vi "Modify Pump Parameters.vi"(6 "timeout (1000 ms)":i32=1000, 7 "Query? (T)":bool=TRUE, 8 "error in (no error)":errorcluster, 10 "Parameters":T1={"Kc"=1.0, "Ti"=0.1, "Td"=0.0, "Min Speed"=0.0, "Max Speed"=100.0}, 11 "Pump in":refnum<class "Pump.lvclass">) -> (0 "error out":errorcluster, 2 "Parameters set":T1={"Kc"=1.0, "Ti"=0.1, "Td"=0.0, "Min Speed"=0.0, "Max Speed"=100.0}, 3 "Pump out":refnum<class "Pump.lvclass">, 4 "timed out?":bool)   [LabVIEW 2014, in "Pump.lvclass"]
doc: "For polynomial coefficients = [a, b, c]\nP(x) = a + b*(x^1) + c*(x^2)"
uses:
  Pump.lvclass
  Parameters - cluster.ctl
  Parameters Payload -- cluster.ctl
  Pump.lvclass/Pump.ctl
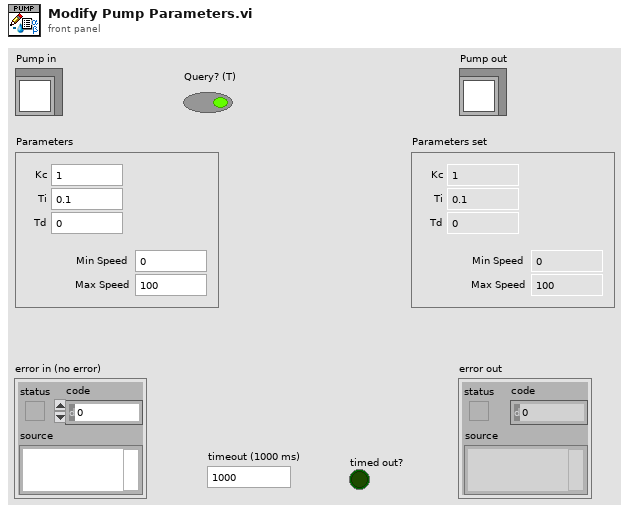
[diagram p1: front panel]
types:
  T1 = typedef "Pump.lvclass/Parameters - cluster.ctl" = cluster{"Kc":dbl, "Ti":dbl, "Td":dbl, "Min Speed":dbl, "Max Speed":dbl}
  T2 = typedef "Pump.lvclass/Parameters Payload -- cluster.ctl" = cluster{"Parameters":T1, "notifier":refnum<notifier>, "Query (T)":bool}
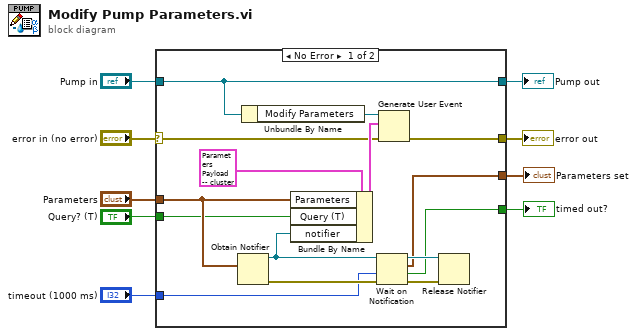
[diagram p0: block diagram]
diagram:
  n1 = case shown="No Error" "error in (no error)" {
    selector: "error in (no error)" -> [w16 w26]
    tunnel: [w15 w26] -> w8
    tunnel: [w19 w25] -> w6
    tunnel: "Pump in" -> [w19 w25]
    tunnel: "timeout (1000 ms)" -> [w23 _]
    tunnel: [w20 _] -> w4
    tunnel: "Parameters" -> [w12 _]
    tunnel: [w14 _] -> w2
    tunnel: "Query? (T)" -> [w10 _]
    frame No Error {
      n2 = Obtain Notifier(notification data type=w12) -> (notifier out=w11:refnum<notifier>, error out=w24:errorcluster)  [unwired: 3 in, 1 out]
      n3 = Unbundle By Name(w19) -> ("Modify Parameters"=w18:refnum<user-event>)
      n4 = Bundle By Name(cluster=T2 {"Parameters"={"Kc"=1.0, "Ti"=0.1, "Td"=0.0, "Min Speed"=0.0, "Max Speed"=100.0}, "notifier"=refnum, "Query (T)"=TRUE} ("Parameters Payload"), "Parameters"=w12, "Query (T)"=w10, "notifier"=w11) -> (w17:T2)
      n5 = Wait on Notification(notifier=w11, timeout in ms (-1)=w23, error in (no error)=w24) -> (notifier out=w22:refnum<notifier>, notification=w20:T1, timed out?=w14:bool, error out=w21:errorcluster)  [unwired: 1 in]
      n6 = Generate User Event(user event=w18, event data cluster=w17, error in=w16) -> (error out=w15:errorcluster)  [unwired: 1 in, 1 out]
      n7 = Release Notifier(notifier=w22, error in (no error)=w21) -> ()  [unwired: 1 in, 3 out]
    }
    frame Error {
    }
  }
  "error out" <- w8
  "Pump out" <- w6
  "Parameters set" <- w4
  "timed out?" <- w2
